vi "BNC555.contents.vi"   [LabVIEW 2014, in "BNC555.lvlib"]
uses:
  BNC555.lvlib
panel:
  # "This is the contens.vi for the BNC555 class."
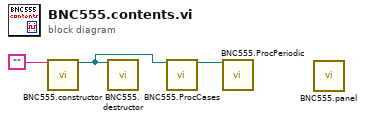
[diagram p0: block diagram]
diagram:
  n1 = call "BNC555.constructor.vi"("name"="") -> ("i ref out"=w1:refnum<vi>)  [unwired: 16 in, 2 out]
  n2 = call "BNC555.destructor.vi"("i ref in"=w1) -> ()  [unwired: 18 in, 1 out]
  n3 = call "BNC555.ProcCases.vi"("i ref in"=w1) -> ("i ref out"=w3:refnum<vi>)  [unwired: 16 in, 2 out]
  n4 = call "BNC555.ProcPeriodic.vi"("i ref in"=w3) -> ()  [unwired: 16 in, 3 out]
  n5 = call "BNC555.panel.vi"() -> ()  [unwired: 19 in, 1 out]
